vi "CteConfig.vi"(8 "error in (no error)":errorcluster, 11 "Cte in":sgl[](array[numeric])) -> (0 "error out":errorcluster, 3 "Cte":sgl[](array[numeric]))   [LabVIEW 2014, in "MathLoop.lvlib"]
doc: "Configura las Constantes."
uses:
  MathLoop.lvlib
panel:
  in  "Stop Cte":bool
  in  "Delete Cte":bool
  in  "Add Cte":bool
  in  "Constantes":i32(listbox)
  in  "Cancel Cte":bool
  in  "Save Cte":bool
  in  "Valor:":sgl format="%.6f"
  in  "Edit Cte":bool
  out "Nro Const:":string="A1"
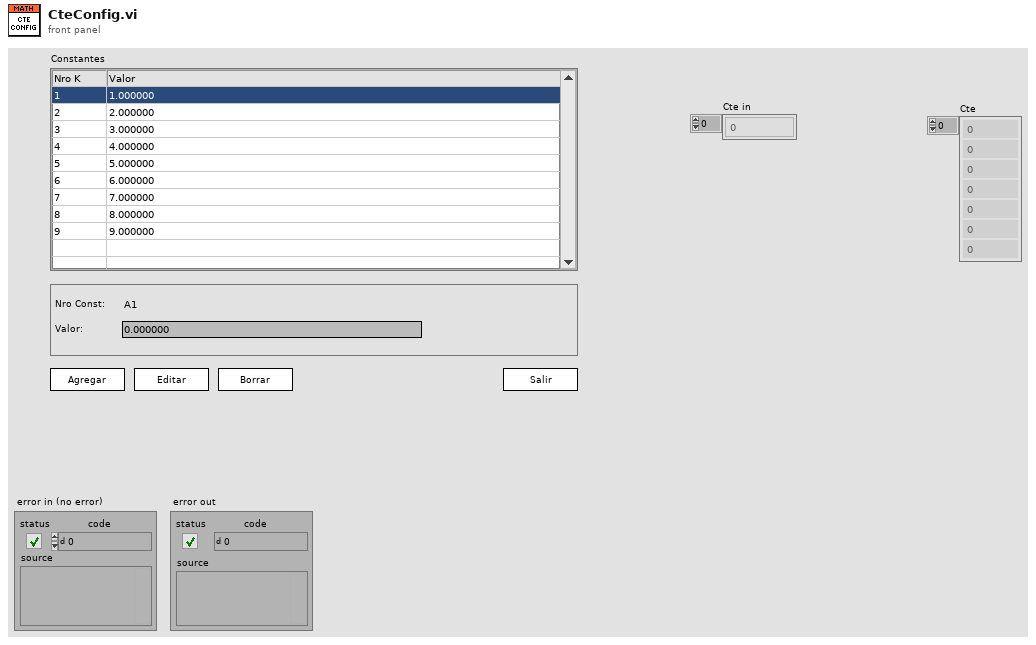
[diagram p1: front panel]
types:
  T1 = enum8{"Enabled", "Disabled", "Disabled and Grayed Out"}
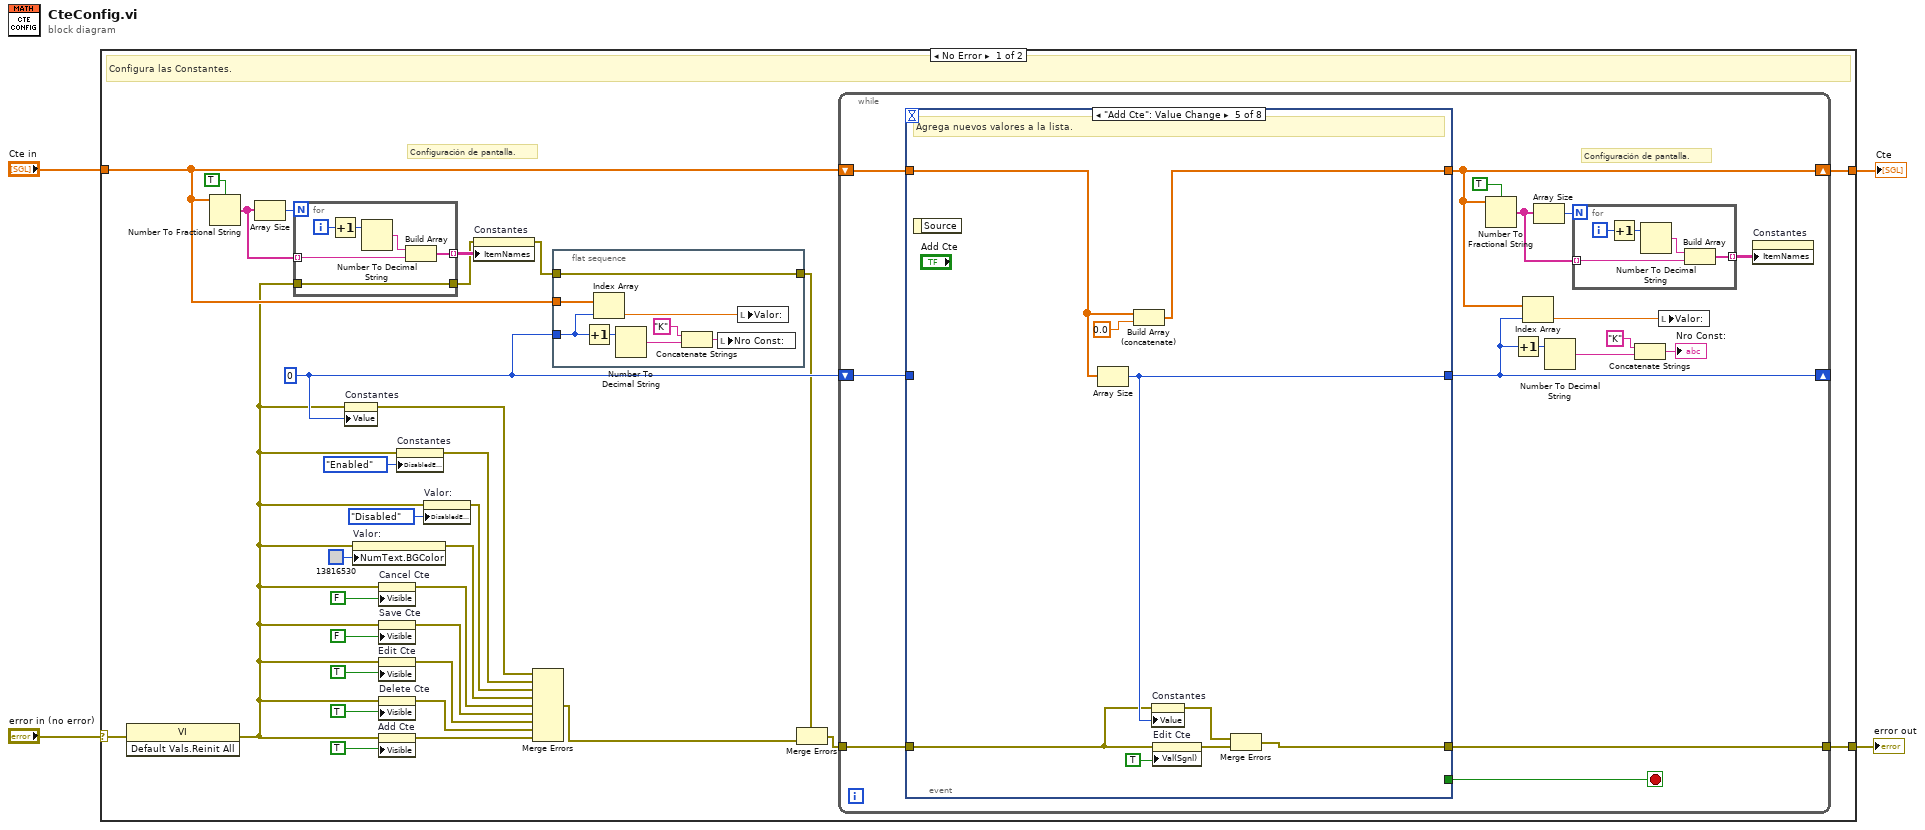
[diagram p0: block diagram]
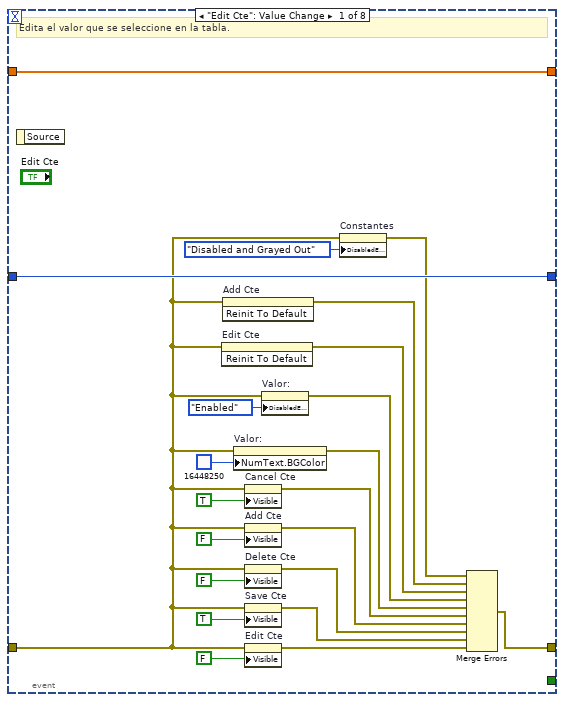
[diagram p2: hidden frame]
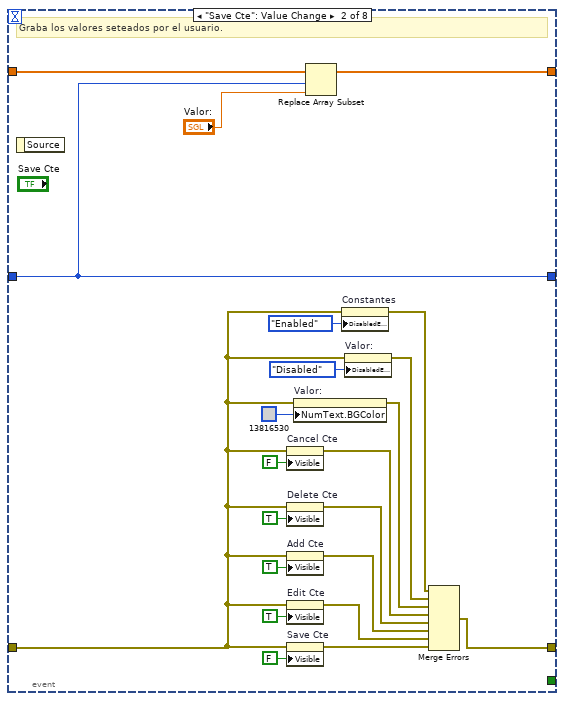
[diagram p3: hidden frame]
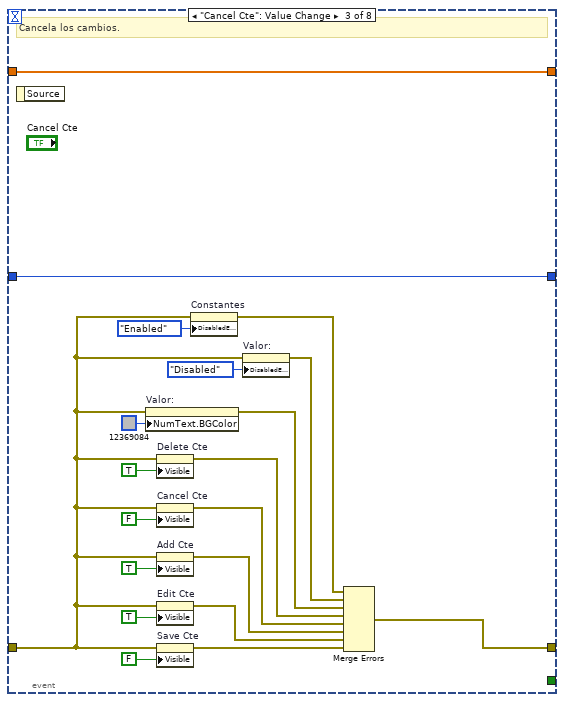
[diagram p4: hidden frame]
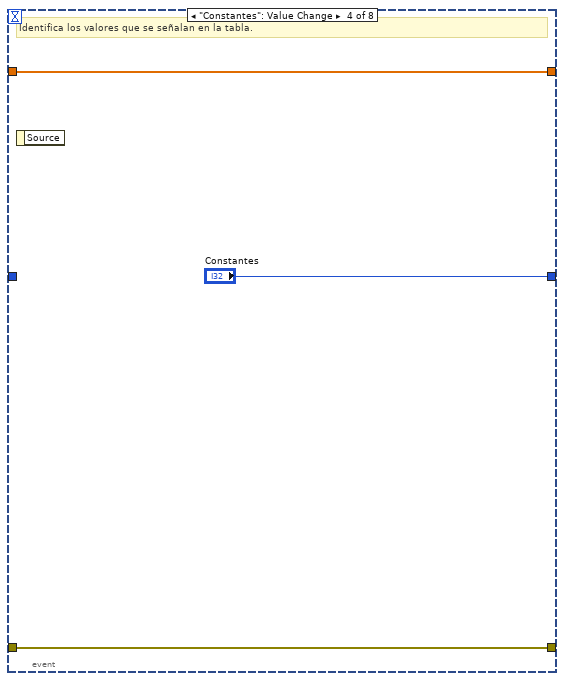
[diagram p5: hidden frame]
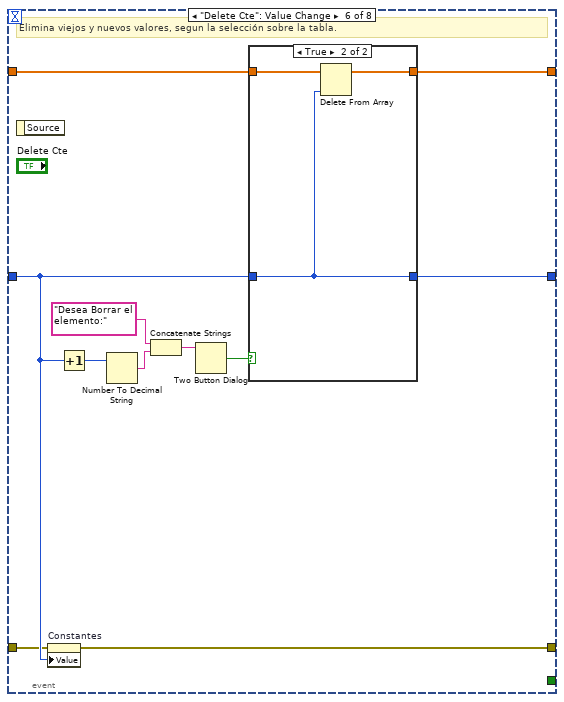
[diagram p6: hidden frame]
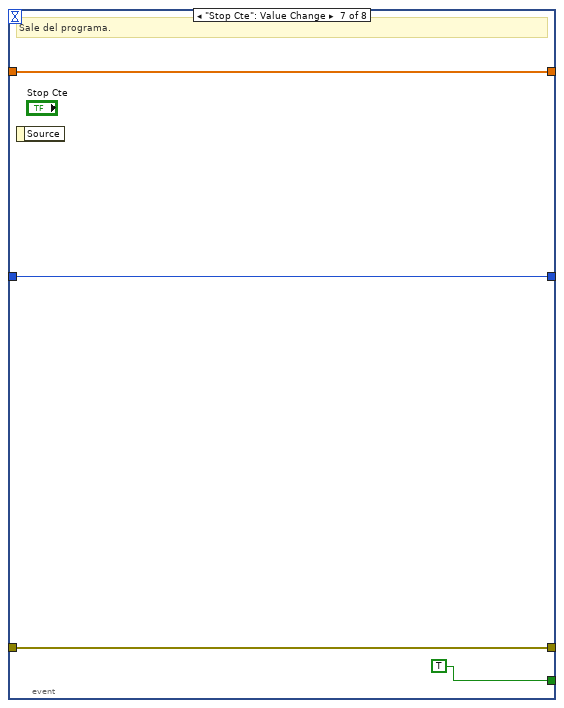
[diagram p8: hidden frame]
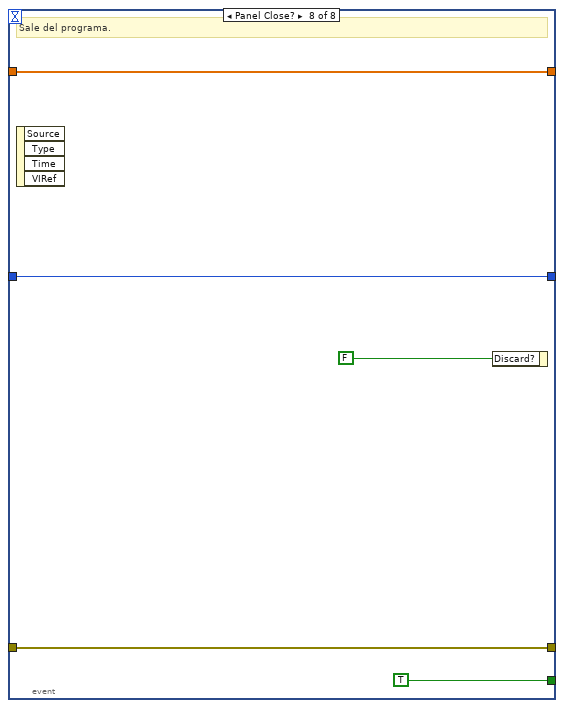
[diagram p9: hidden frame]
diagram:
  n1 = case shown="No Error" "error in (no error)" {
    selector: "error in (no error)" -> [w5 w173]
    tunnel: [w36 w173] -> w4
    tunnel: [w21 w174] -> w3
    tunnel: "Cte in" -> [w16 w174]
    frame No Error {
      w15 = 0 ("disabled index (col)")
      # "Configuración de pantalla."
      # "Configura las Constantes."
      n2 = invoke class="VI" method="Default Vals.Reinit All"(error in=w5) -> (error out=w6:errorcluster)  [unwired: 2 in, 2 out]
      n3 = Number To Fractional String(use system decimal point (T)=TRUE, number=w16) -> (F-format string=w20:string[])  [unwired: 2 in]
      n4 = Array Size(array=w20) -> (size(s)=w30:i32)
      n5 = for {
        N: w30 -> [_]
        tunnel: w20 -> [w50] mode=indexing
        tunnel: [w48] -> w29 mode=indexing
        tunnel: w6 -> [w45]
        tunnel: [w45] -> w14
        i -> [w46]
        n6 = Increment(x=w46) -> (x+1=w47:i32)
        n7 = Number To Decimal String(number=w47) -> (decimal integer string=w49:string)  [unwired: 1 in]
        n8 = Build Array(w49, w50) -> (w48:string[])
      }
      n9 = property on="Constantes" class="MCListbox (strict)"(error in=w6, "Value"=w15) -> (error out=w7:errorcluster)  [unwired: 1 in, 1 out]
      n10 = property on="Valor:" class="DigNum (strict)"(error in=w6, "NumText.BGColor"=u32 13816530) -> (error out=w27:errorcluster)  [unwired: 1 in, 1 out]
      n11 = property on="Cancel Cte" class="Bool"(error in=w6, "Visible"=FALSE) -> (error out=w26:errorcluster)  [unwired: 1 in, 1 out]
      n12 = property on="Save Cte" class="Bool"(error in=w6, "Visible"=FALSE) -> (error out=w33:errorcluster)  [unwired: 1 in, 1 out]
      n13 = property on="Edit Cte" class="Bool (strict)"(error in=w6, "Visible"=TRUE) -> (error out=w32:errorcluster)  [unwired: 1 in, 1 out]
      n14 = property on="Delete Cte" class="Bool"(error in=w6, "Visible"=TRUE) -> (error out=w24:errorcluster)  [unwired: 1 in, 1 out]
      n15 = property on="Add Cte" class="Bool (strict)"(error in=w6, "Visible"=TRUE) -> (error out=w22:errorcluster)  [unwired: 1 in, 1 out]
      n16 = property on="Constantes" class="MCListbox (strict)"(error in=w6, "DisabledEnum"=T1."Enabled" ("Disabled")) -> (error out=w8:errorcluster)  [unwired: 1 in, 1 out]
      n17 = property on="Valor:" class="DigNum (strict)"(error in=w6, "DisabledEnum"=T1."Disabled" ("Disabled")) -> (error out=w17:errorcluster)  [unwired: 1 in, 1 out]
      n18 = property on="Constantes" class="MCListbox (strict)"(error in=w14, "ItemNames"=w29) -> (error out=w13:errorcluster)  [unwired: 1 in, 1 out]
      n19 = Merge Errors(w7, w8, w17, w27, w26, w33, w32, w24, w22) -> (w12:errorcluster)
      n20 = flat-sequence {
        tunnel: w16 -> [w39]
        tunnel: w15 -> [w38]
        tunnel: w13 -> [w37]
        tunnel: [w37] -> w10
        frame #0 {
          n21 = Increment(x=w38) -> (x+1=w43:i32)
          n22 = Index Array(array=w39, index=w38) -> (element=w41:sgl)
          n23 = Number To Decimal String(number=w43) -> (decimal integer string=w44:string)  [unwired: 1 in]
          n24 = Concatenate Strings("K" ("string"), w44) -> (w40:string)
          n25 = local write "Nro Const:"(w40) -> ()
          n26 = local write "Valor:"(w41) -> ()
        }
      }
      n27 = Merge Errors(w10, w12) -> (w11:errorcluster)
      n28 = while {
        shift-right: [w52] -> w21
        shift-left: w16 -> [w63]
        shift-right: [w61] -> _
        shift-left: w15 -> [w62]
        tunnel: w11 -> [w66]
        tunnel: [w65] -> w36
        stop <- w64 stop-if-true
        # "Configuración de pantalla."
        n29 = event shown="[4] \"Add Cte\": Value Change" {
          selector: _ -> [_ _ _ _ _ _ _ _]
          dyn-events: _ -> [_ _ _ _ _ _ _ _]
          timeout: _ -> [_ _ _ _ _ _ _ _]
          tunnel: w63 -> [w87 w108 w135 w138 w144 w156 w166 w172]
          tunnel: [w87 w107 w135 w138 w147 w155 w166 w172] -> w52
          tunnel: [w86 w109 w134 "Constantes" w143 w157 w165 w171] -> w61
          tunnel: w62 -> [w86 w109 w134 _ _ w150 w165 w171]
          tunnel: w66 -> [w72 w94 w116 w136 w140 w149 w167 w170]
          tunnel: [w88 w110 w126 w136 w139 w148 w167 w170] -> w65
          tunnel: [_ _ _ _ _ _ TRUE TRUE] -> w64
          event "Edit Cte": Value Change {
            # "Edita el valor que se seleccione en la tabla."
            n30 = event-data() -> ()  [unwired: 1 in, 1 out]
            n31 = invoke on="Edit Cte" class="Bool (strict)" method="Reinit To Default"(error in=w72) -> (error out=w76:errorcluster)  [unwired: 2 in, 2 out]
            n32 = invoke on="Add Cte" class="Bool (strict)" method="Reinit To Default"(error in=w72) -> (error out=w77:errorcluster)  [unwired: 2 in, 2 out]
            n33 = property on="Valor:" class="DigNum (strict)"(error in=w72, "NumText.BGColor"=u32 16448250) -> (error out=w80:errorcluster)  [unwired: 1 in, 1 out]
            n34 = property on="Cancel Cte" class="Bool"(error in=w72, "Visible"=TRUE) -> (error out=w79:errorcluster)  [unwired: 1 in, 1 out]
            n35 = property on="Add Cte" class="Bool (strict)"(error in=w72, "Visible"=FALSE) -> (error out=w82:errorcluster)  [unwired: 1 in, 1 out]
            n36 = property on="Delete Cte" class="Bool"(error in=w72, "Visible"=FALSE) -> (error out=w84:errorcluster)  [unwired: 1 in, 1 out]
            n37 = property on="Save Cte" class="Bool"(error in=w72, "Visible"=TRUE) -> (error out=w89:errorcluster)  [unwired: 1 in, 1 out]
            n38 = property on="Edit Cte" class="Bool (strict)"(error in=w72, "Visible"=FALSE) -> (error out=w93:errorcluster)  [unwired: 1 in, 1 out]
            n39 = property on="Valor:" class="DigNum (strict)"(error in=w72, "DisabledEnum"=T1."Enabled" ("Disabled")) -> (error out=w75:errorcluster)  [unwired: 1 in, 1 out]
            n40 = property on="Constantes" class="MCListbox (strict)"(error in=w72, "DisabledEnum"=T1."Disabled and Grayed Out" ("Disabled")) -> (error out=w73:errorcluster)  [unwired: 1 in, 1 out]
            n41 = Merge Errors(w73, w77, w76, w75, w80, w79, w82, w84, w89, w93) -> (w88:errorcluster)
          }
          event "Save Cte": Value Change {
            # "Graba los valores seteados por el usuario."
            n42 = event-data() -> ()  [unwired: 1 in, 1 out]
            n43 = property on="Cancel Cte" class="Bool"(error in=w94, "Visible"=FALSE) -> (error out=w102:errorcluster)  [unwired: 1 in, 1 out]
            n44 = property on="Delete Cte" class="Bool"(error in=w94, "Visible"=TRUE) -> (error out=w101:errorcluster)  [unwired: 1 in, 1 out]
            n45 = property on="Add Cte" class="Bool (strict)"(error in=w94, "Visible"=TRUE) -> (error out=w105:errorcluster)  [unwired: 1 in, 1 out]
            n46 = property on="Edit Cte" class="Bool (strict)"(error in=w94, "Visible"=TRUE) -> (error out=w115:errorcluster)  [unwired: 1 in, 1 out]
            n47 = property on="Save Cte" class="Bool"(error in=w94, "Visible"=FALSE) -> (error out=w114:errorcluster)  [unwired: 1 in, 1 out]
            n48 = property on="Valor:" class="DigNum (strict)"(error in=w94, "NumText.BGColor"=u32 13816530) -> (error out=w100:errorcluster)  [unwired: 1 in, 1 out]
            n49 = Replace Array Subset(array=w108, new element="Valor:", index=w109) -> (w107:sgl[])
            n50 = property on="Constantes" class="MCListbox (strict)"(error in=w94, "DisabledEnum"=T1."Enabled" ("Disabled")) -> (error out=w95:errorcluster)  [unwired: 1 in, 1 out]
            n51 = property on="Valor:" class="DigNum (strict)"(error in=w94, "DisabledEnum"=T1."Disabled" ("Disabled")) -> (error out=w97:errorcluster)  [unwired: 1 in, 1 out]
            n52 = Merge Errors(w95, w97, w100, w102, w101, w105, w115, w114) -> (w110:errorcluster)
          }
          event "Cancel Cte": Value Change {
            # "Cancela los cambios."
            n53 = event-data() -> ()  [unwired: 1 in, 1 out]
            n54 = property on="Valor:" class="DigNum (strict)"(error in=w116, "NumText.BGColor"=u32 12369084) -> (error out=w123:errorcluster)  [unwired: 1 in, 1 out]
            n55 = property on="Delete Cte" class="Bool"(error in=w116, "Visible"=TRUE) -> (error out=w122:errorcluster)  [unwired: 1 in, 1 out]
            n56 = property on="Cancel Cte" class="Bool"(error in=w116, "Visible"=FALSE) -> (error out=w121:errorcluster)  [unwired: 1 in, 1 out]
            n57 = property on="Add Cte" class="Bool (strict)"(error in=w116, "Visible"=TRUE) -> (error out=w127:errorcluster)  [unwired: 1 in, 1 out]
            n58 = property on="Edit Cte" class="Bool (strict)"(error in=w116, "Visible"=TRUE) -> (error out=w133:errorcluster)  [unwired: 1 in, 1 out]
            n59 = property on="Save Cte" class="Bool"(error in=w116, "Visible"=FALSE) -> (error out=w132:errorcluster)  [unwired: 1 in, 1 out]
            n60 = property on="Constantes" class="MCListbox (strict)"(error in=w116, "DisabledEnum"=T1."Enabled" ("Disabled")) -> (error out=w117:errorcluster)  [unwired: 1 in, 1 out]
            n61 = property on="Valor:" class="DigNum (strict)"(error in=w116, "DisabledEnum"=T1."Disabled" ("Disabled")) -> (error out=w119:errorcluster)  [unwired: 1 in, 1 out]
            n62 = Merge Errors(w117, w119, w123, w122, w121, w127, w133, w132) -> (w126:errorcluster)
          }
          event "Constantes": Value Change {
            # "Identifica los valores que se señalan en la tabla."
            n63 = event-data() -> ()  [unwired: 1 in, 1 out]
          }
          event "Add Cte": Value Change {
            # "Agrega nuevos valores a la lista."
            n64 = event-data() -> ()  [unwired: 1 in, 1 out]
            n65 = Array Size(array=w144) -> (size(s)=w143:i32)
            n66 = Build Array (concatenate)(w144, sgl 0.0) -> (w147:sgl[])
            n67 = property on="Constantes" class="MCListbox (strict)"(error in=w140, "Value"=w143) -> (error out=w142:errorcluster)  [unwired: 1 in, 1 out]
            n68 = property on="Edit Cte" class="Bool (strict)"(error in=w140, "Val(Sgnl)"=TRUE) -> (error out=w141:errorcluster)  [unwired: 1 in, 1 out]
            n69 = Merge Errors(w142, w141) -> (w139:errorcluster)
          }
          event "Delete Cte": Value Change {
            # "Elimina viejos y nuevos valores, segun la selección sobre la tabla."
            n70 = event-data() -> ()  [unwired: 1 in, 1 out]
            n71 = property on="Constantes" class="MCListbox (strict)"(error in=w149, "Value"=w150) -> (error out=w148:errorcluster)  [unwired: 1 in, 1 out]
            n72 = Increment(x=w150) -> (x+1=w151:i32)
            n73 = Number To Decimal String(number=w151) -> (decimal integer string=w153:string)  [unwired: 1 in]
            n74 = Concatenate Strings("Desea Borrar el elemento:" ("message"), w153) -> (w152:string)
            n75 = Two Button Dialog(message=w152) -> (T button?=w158:bool)  [unwired: 2 in]
            n76 = case shown="True" w158 {
              tunnel: w156 -> [w159 w163]
              tunnel: [w160 w161] -> w157
              tunnel: w150 -> [w160 w161]
              tunnel: [w159 w162] -> w155
              frame False {
              }
              frame True {
                n77 = Delete From Array(array=w163, index=w161) -> (array with subset deleted=w162:sgl[])  [unwired: 1 in, 1 out]
              }
            }
          }
          event "Stop Cte": Value Change {
            # "Sale del programa."
            n78 = event-data() -> ()  [unwired: 1 in, 1 out]
          }
          event Panel Close? {
            # "Sale del programa."
            n79 = event-data() -> ()  [unwired: 1 in, 4 out]
            n80 = event-data("Discard?"=FALSE) -> ()  [unwired: 1 in, 1 out]
          }
        }
        n81 = Number To Fractional String(use system decimal point (T)=TRUE, number=w52) -> (F-format string=w51:string[])  [unwired: 2 in]
        n82 = Increment(x=w61) -> (x+1=w57:i32)
        n83 = Index Array(array=w52, index=w61) -> (element=w54:sgl)
        n84 = Array Size(array=w51) -> (size(s)=w60:i32)
        n85 = Number To Decimal String(number=w57) -> (decimal integer string=w58:string)  [unwired: 1 in]
        n86 = for {
          N: w60 -> [_]
          tunnel: w51 -> [w71] mode=indexing
          tunnel: [w69] -> w59 mode=indexing
          i -> [w67]
          n87 = Increment(x=w67) -> (x+1=w68:i32)
          n88 = Number To Decimal String(number=w68) -> (decimal integer string=w70:string)  [unwired: 1 in]
          n89 = Build Array(w70, w71) -> (w69:string[])
        }
        n90 = Concatenate Strings("K" ("string"), w58) -> (→"Nro Const:":string)
        n91 = local write "Valor:"(w54) -> ()
        n92 = property on="Constantes" class="MCListbox (strict)"("ItemNames"=w59) -> ()  [unwired: 2 in, 2 out]
      }
    }
    frame Error {
    }
  }
  "error out" <- w4
  "Cte" <- w3
